vi "module-12-analog-pid-complex.vi"() -> ()   [LabVIEW 2019]
uses:
  <vilib>/Rock Robotics/WPI/ThirdParty/JAS_Junk/TrajLib/PID_CONTROLLER.ctl
  <vilib>/Rock Robotics/WPI/ThirdParty/JAS_Junk/TrajLib/LinearFilter_ResetToValue.vi
  <vilib>/Rock Robotics/WPI/ThirdParty/JAS_Junk/TrajLib/LinearFilter_Calculate.vi
  <vilib>/Rock Robotics/WPI/ThirdParty/JAS_Junk/TrajLib/PIDController_AtSetpoint.vi
  <vilib>/Rock Robotics/WPI/ThirdParty/JAS_Junk/TrajLib/PIDController_SetPIDF.vi
  <vilib>/Rock Robotics/WPI/ThirdParty/JAS_Junk/TrajLib/PIDController_SetDerivativeFilter.vi
  <vilib>/Rock Robotics/WPI/ThirdParty/JAS_Junk/TrajLib/PIDController_SetIntegratorRange.vi
  <vilib>/Rock Robotics/WPI/ThirdParty/JAS_Junk/TrajLib/PIDController_SetTolerancePandV.vi
  <vilib>/Rock Robotics/WPI/ThirdParty/JAS_Junk/TrajLib/PIDController_DisableContinousInput.vi
  <vilib>/Rock Robotics/WPI/ThirdParty/JAS_Junk/TrajLib/PIDController_EnableContinousInput.vi
  <vilib>/Rock Robotics/WPI/ThirdParty/JAS_Junk/TrajLib/PIDController_Reset.vi
  <vilib>/Rock Robotics/WPI/ThirdParty/JAS_Junk/TrajLib/PIDController_New.vi
  <vilib>/Rock Robotics/WPI/ThirdParty/JAS_Junk/TrajLib/PIDController_SetOutputLimits.vi
  <vilib>/Rock Robotics/WPI/ThirdParty/JAS_Junk/TrajLib/ControllerUtil_GetModulusError.vi
  <vilib>/Rock Robotics/WPI/ThirdParty/JAS_Junk/TrajLib/PIDController_NewPeriod.vi
  <vilib>/Rock Robotics/SystemInterfaces/NetworkCommunication/NetComm_UsageReport_report.vi
  <vilib>/addons/control/pid/pid.llb/PID Lead-Lag (DBL).vi
  <vilib>/Rock Robotics/WPI/ThirdParty/JAS_Junk/TrajLib/Util_LibraryGlobals.vi
  <vilib>/Rock Robotics/WPI/ThirdParty/JAS_Junk/TrajLib/PIDController_AdvCalculate_FF_Sp_Pv.vi
  <vilib>/Rock Robotics/WPI/ThirdParty/JAS_Junk/TrajLib/LinearFilter_MovingAverage.vi
  <vilib>/Rock Robotics/WPI/ThirdParty/JAS_Junk/TrajLib/LinearFilter_LowPassBW1.vi
  <vilib>/Rock Robotics/WPI/ThirdParty/JAS_Junk/TrajLib/LinearFilter_LowPassBW2.vi
  <vilib>/Rock Robotics/WPI/ThirdParty/JAS_Junk/TrajLib/LinearFilter_HighPassBW1.vi
  <vilib>/Rock Robotics/WPI/ThirdParty/JAS_Junk/TrajLib/LinearFilter_HighPassBW2.vi
  <vilib>/addons/control/pid/NI_PID_pid.lvlib
  <vilib>/Rock Robotics/WPI/ThirdParty/JAS_Junk/TrajLib/Trajectory_Library.lvlib
panel:
  in  "Tab Control":T1(tab)
  in  "Enable Noise":bool=TRUE
  in  "Auto / Manual":bool=TRUE
  out "Selected Speed Demand":dbl format="%10.2f"
  in  "Desired Speed":dbl(slide)=-0.22222222222222499 scale=-50.0..50.0 scale format="%#.1f"
  out "Selected Speed Target":dbl format="%10.2f"
  out "Right Motor Demand":dbl format="%11.3f"
  out "Right Wheel Speed":dbl(knob)=-2.895988890827539e-05 scale=-60.0..60.0
  out "Right Wheel Error":dbl format="%11.3f"
  out "Right Wheel Speed":dbl format="%10.2f"
  out "Left Wheel Speed":dbl(knob)=-2.895988890827539e-05 scale=-60.0..60.0
  out "Left Wheel Error":dbl format="%11.3f"
  out "Left Motor Demand":dbl format="%11.3f"
  out "Left Wheel Speed":dbl format="%10.2f"
  in  "MinOutput 2":dbl=-9.9e+32
  in  "MaxOutput 2":dbl=9.9e+32
  in  "MinInput 2":dbl
  in  "MaxInput 2":dbl
  in  "MinOutput":dbl=-9.9e+32
  in  "MaxOutput":dbl=9.9e+32
  in  "MinInput":dbl
  in  "MaxInput":dbl
  in  "SetPoint Change Rate":dbl=80.0 min=1.0 max=9000.0 format="%14.4f"
  in  "Right-Kp":dbl=0.12
  in  "Right-Ki":dbl=1.2
  in  "Right-Kd":dbl
  in  "Right-Max-I":dbl=1.0
  in  "Right-Min-I":dbl=-1.0
  in  "Right-Kf":dbl=0.02
  in  "Left-Kp":dbl=0.12
  in  "Left-Ki":dbl=1.2
  in  "Left-Kd":dbl
  in  "Left-Max-I":dbl=1.0
  in  "Left-Min-I":dbl=-1.0
  in  "Left-Kf":dbl=0.02
  out "Right-PID Data":T2={"Kp"=0.0, "Ki"=0.0, "Kd"=0.0, "Period"=0.0, "Max_Integral"=0.0, "Min_Integral"=0.0, "Max_Input"=0.0, "Min_Input"=0.0, "Continuous"=FALSE, "PositionError"=0.0, "VelocityError"=0.0, "PrevError"=0.0, "TotalError"=0.0, "PositionTolerance"=0.0, "VelocityTolerance"=0.0, "SetPoint"=0.0, "Kf"=0.0, "Prev_Deriv"=0.0, "Prev_Deriv 2"=0.0, "DerivativeFilter"=FALSE, "Min_Output"=-9.99e+35, "Max_Output"=9.9e+35, "Prev_F_P"=0.0, "Prev_F_P_2"=0.0, "AntiWindupActive"=FALSE, "Measurement"=0.0} {"Measurement" format="%16_6e"; "Prev_F_P_2" format="%16_6e"; "Prev_F_P" format="%16_6e"; "Max_Output" format="%16_6e"; "Min_Output" format="%16_6e"; "Prev_Deriv 2" format="%16_6e"; "Prev_Deriv" format="%16_6e"; "Kf" format="%16_6e"; "SetPoint" format="%16_6e"; "VelocityTolerance" format="%16_6e"; "PositionTolerance" format="%16_6e"; "TotalError" format="%16_6e"; "PrevError" format="%16_6e"; "VelocityError" format="%16_6e"; "PositionError" format="%16_6e"; "Min_Input" format="%16_6e"; "Max_Input" format="%16_6e"; "Min_Integral" format="%16_6e"; "Max_Integral" format="%16_6e"; "Period" format="%16_6e"; "Kd" format="%16_6e"; "Ki" format="%16_6e"; "Kp" format="%16_6e"}
  out "Left-PID Data":T2={"Kp"=0.0, "Ki"=0.0, "Kd"=0.0, "Period"=0.0, "Max_Integral"=0.0, "Min_Integral"=0.0, "Max_Input"=0.0, "Min_Input"=0.0, "Continuous"=FALSE, "PositionError"=0.0, "VelocityError"=0.0, "PrevError"=0.0, "TotalError"=0.0, "PositionTolerance"=0.0, "VelocityTolerance"=0.0, "SetPoint"=0.0, "Kf"=0.0, "Prev_Deriv"=0.0, "Prev_Deriv 2"=0.0, "DerivativeFilter"=FALSE, "Min_Output"=-9.99e+35, "Max_Output"=9.9e+35, "Prev_F_P"=0.0, "Prev_F_P_2"=0.0, "AntiWindupActive"=FALSE, "Measurement"=0.0} {"Measurement" format="%16_6e"; "Prev_F_P_2" format="%16_6e"; "Prev_F_P" format="%16_6e"; "Max_Output" format="%16_6e"; "Min_Output" format="%16_6e"; "Prev_Deriv 2" format="%16_6e"; "Prev_Deriv" format="%16_6e"; "Kf" format="%16_6e"; "SetPoint" format="%16_6e"; "VelocityTolerance" format="%16_6e"; "PositionTolerance" format="%16_6e"; "TotalError" format="%16_6e"; "PrevError" format="%16_6e"; "VelocityError" format="%16_6e"; "PositionError" format="%16_6e"; "Min_Input" format="%16_6e"; "Max_Input" format="%16_6e"; "Min_Integral" format="%16_6e"; "Max_Integral" format="%16_6e"; "Period" format="%16_6e"; "Kd" format="%16_6e"; "Ki" format="%16_6e"; "Kp" format="%16_6e"}
  in  "RightWheelNoise":dbl
  in  "LeftWheelNoise":dbl
  in  "RightWheelSpeed":dbl
  in  "LeftWheelSpeed":dbl
  in  "RightMotorOutput":dbl
  in  "LeftMotorOutput":dbl
  in  "SpeedSetpoint":dbl
  in  "SpeedTarget":dbl
  in  "SpeedControlEnabled":bool
  out "SP, PV, CO Right":T3(graph)
  out "SP, PV, CO Left":T3(graph)
  # "Example of Closed Loop \nMotor Speed Control"
  # "Enter a desired speed and then press the Set Speed Target \nbutton.  This simulates the joystick input."
  # "This value shows the current speed of each wheel.  This is measured by an encoder.  The encoder measures\n speed by counting pulses of the wheel turning and dividing by the time interval.  Total distance change\nis also a result.  This value is called the \"Process Variable\"."
  # "FT/SEC"
  # "FT/SEC"
  # "FT/SEC"
  # "FT/SEC"
  # "The Speed Target is rate limited so not to make\nto drastic a change in the desired speed.  (This is\nwhat happens mechanically when pushing the gas\npedal of a real car.)"
  # "This error value shows the error between the current speed\nand the speed demand."
  # "FT/SEC"
  # "This example adds a \"Manual\" mode so that the still operates\nif the encoder fails."
  # "FT/SEC"
  # "FT/SEC"
  # "This value shows the current motor output demand.  This could also be a motor speed demand and \nanother closed loop controller would control the motor speed.  In this simple example this value is \nused to drive the simulated motor directly.  This motor demand is called the \"Control Output\"."
  # "Enables some simulated process noise"
  # "FT/SEC/SEC"
  # "These are the tuning parameters for the PID VI"
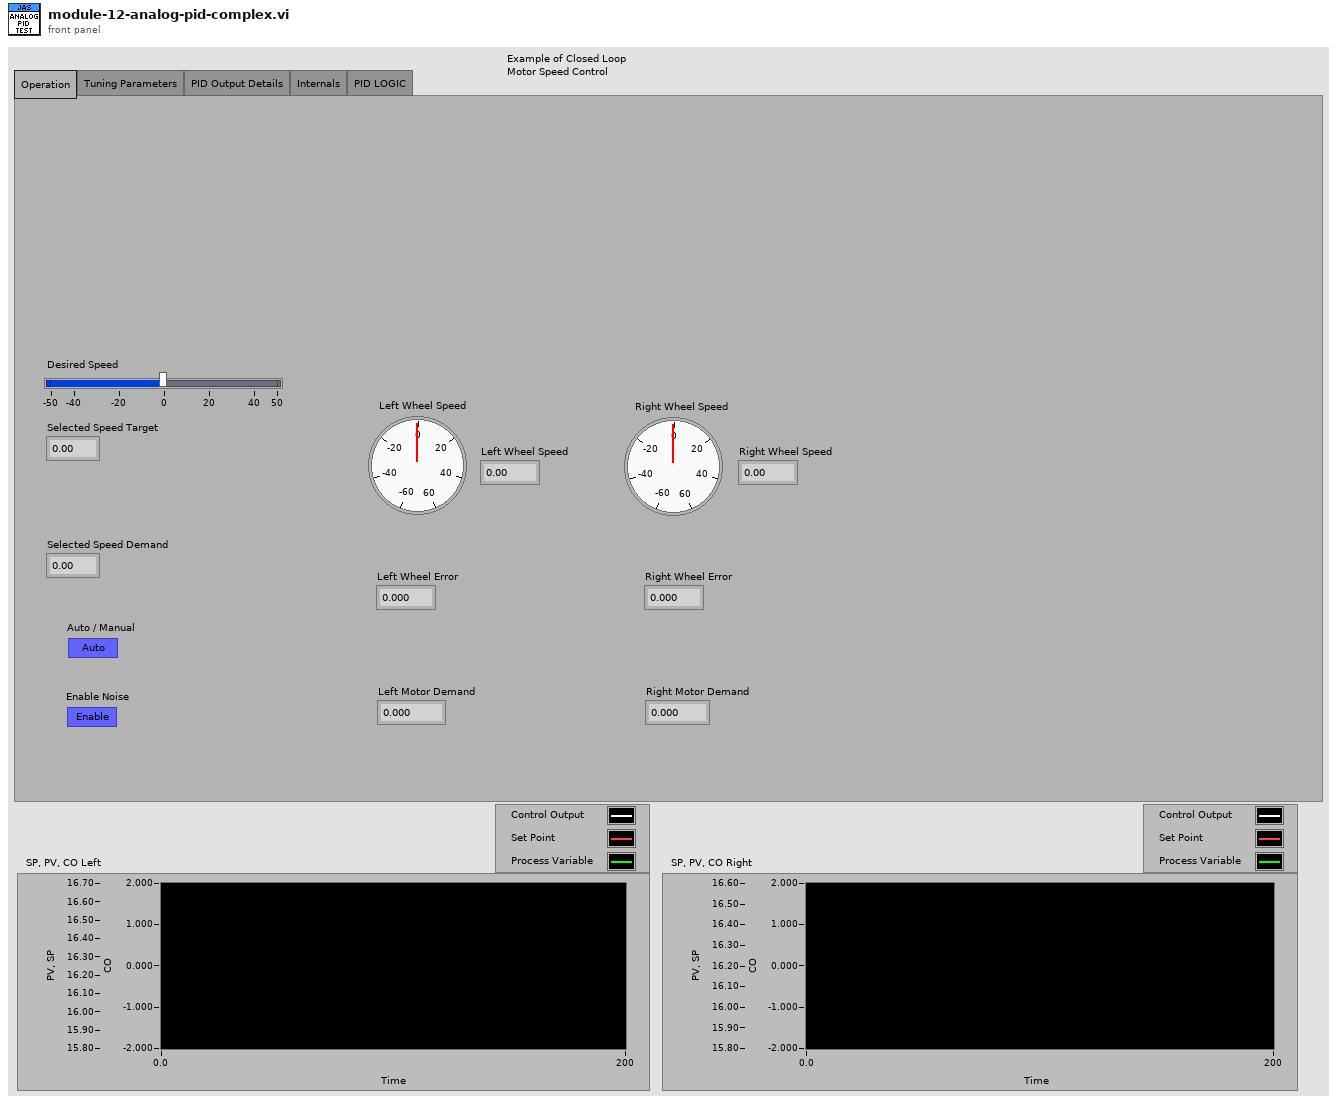
[diagram p1: front panel]
types:
  T1 = enum32{"Operation", "Tuning Parameters", "PID Output Details", "Internals", "PID LOGIC"}
  T2 = typedef "Trajectory_Library.lvlib/PID_CONTROLLER.ctl" = cluster{"Kp":dbl, "Ki":dbl, "Kd":dbl, "Period":dbl, "Max_Integral":dbl, "Min_Integral":dbl, "Max_Input":dbl, "Min_Input":dbl, "Continuous":bool, "PositionError":dbl, "VelocityError":dbl, "PrevError":dbl, "TotalError":dbl, "PositionTolerance":dbl, "VelocityTolerance":dbl, "SetPoint":dbl, "Kf":dbl, "Prev_Deriv":dbl, "Prev_Deriv 2":dbl, "DerivativeFilter":bool, "Min_Output":dbl, "Max_Output":dbl, "Prev_F_P":dbl, "Prev_F_P_2":dbl, "AntiWindupActive":bool, "Measurement":dbl}
  T3 = cluster{"MotorDemand":dbl, "CurrentSetpoint":dbl, "CurrentPosition":dbl}
  T4 = cluster{"gain":dbl, "lag time":dbl, "lead time":dbl}
  T5 = typedef "Trajectory_Library.lvlib/PID_ADV_LIMITS.ctl" = cluster{"MaxInput":dbl, "MinInput":dbl, "Continuous":bool, "MaxOutput":dbl, "MinOutput":dbl}
  T6 = enum16{"Moving Average", "Low Pass 1st Order Butterworth", "Low Pass 2nd Order Butterworth", "High Pass 1st Order Butterworth", "High Pass 2nd Order Butterworth"}
  T7 = cluster{"LeftMotorOutput":dbl, "SpeedSetpoint":dbl, "LeftWheelSpeed":dbl}
  T8 = cluster{"RightMotorOutput":dbl, "SpeedSetpoint":dbl, "RightWheelSpeed":dbl}
  T9 = typedef "Trajectory_Library.lvlib/PID_ADV_TUNING.ctl" = cluster{"Kf":dbl, "Kp":dbl, "Ki":dbl, "Kd":dbl, "MaximumIntegral":dbl, "MinimumIntegral":dbl, "Filter Derivative":bool}
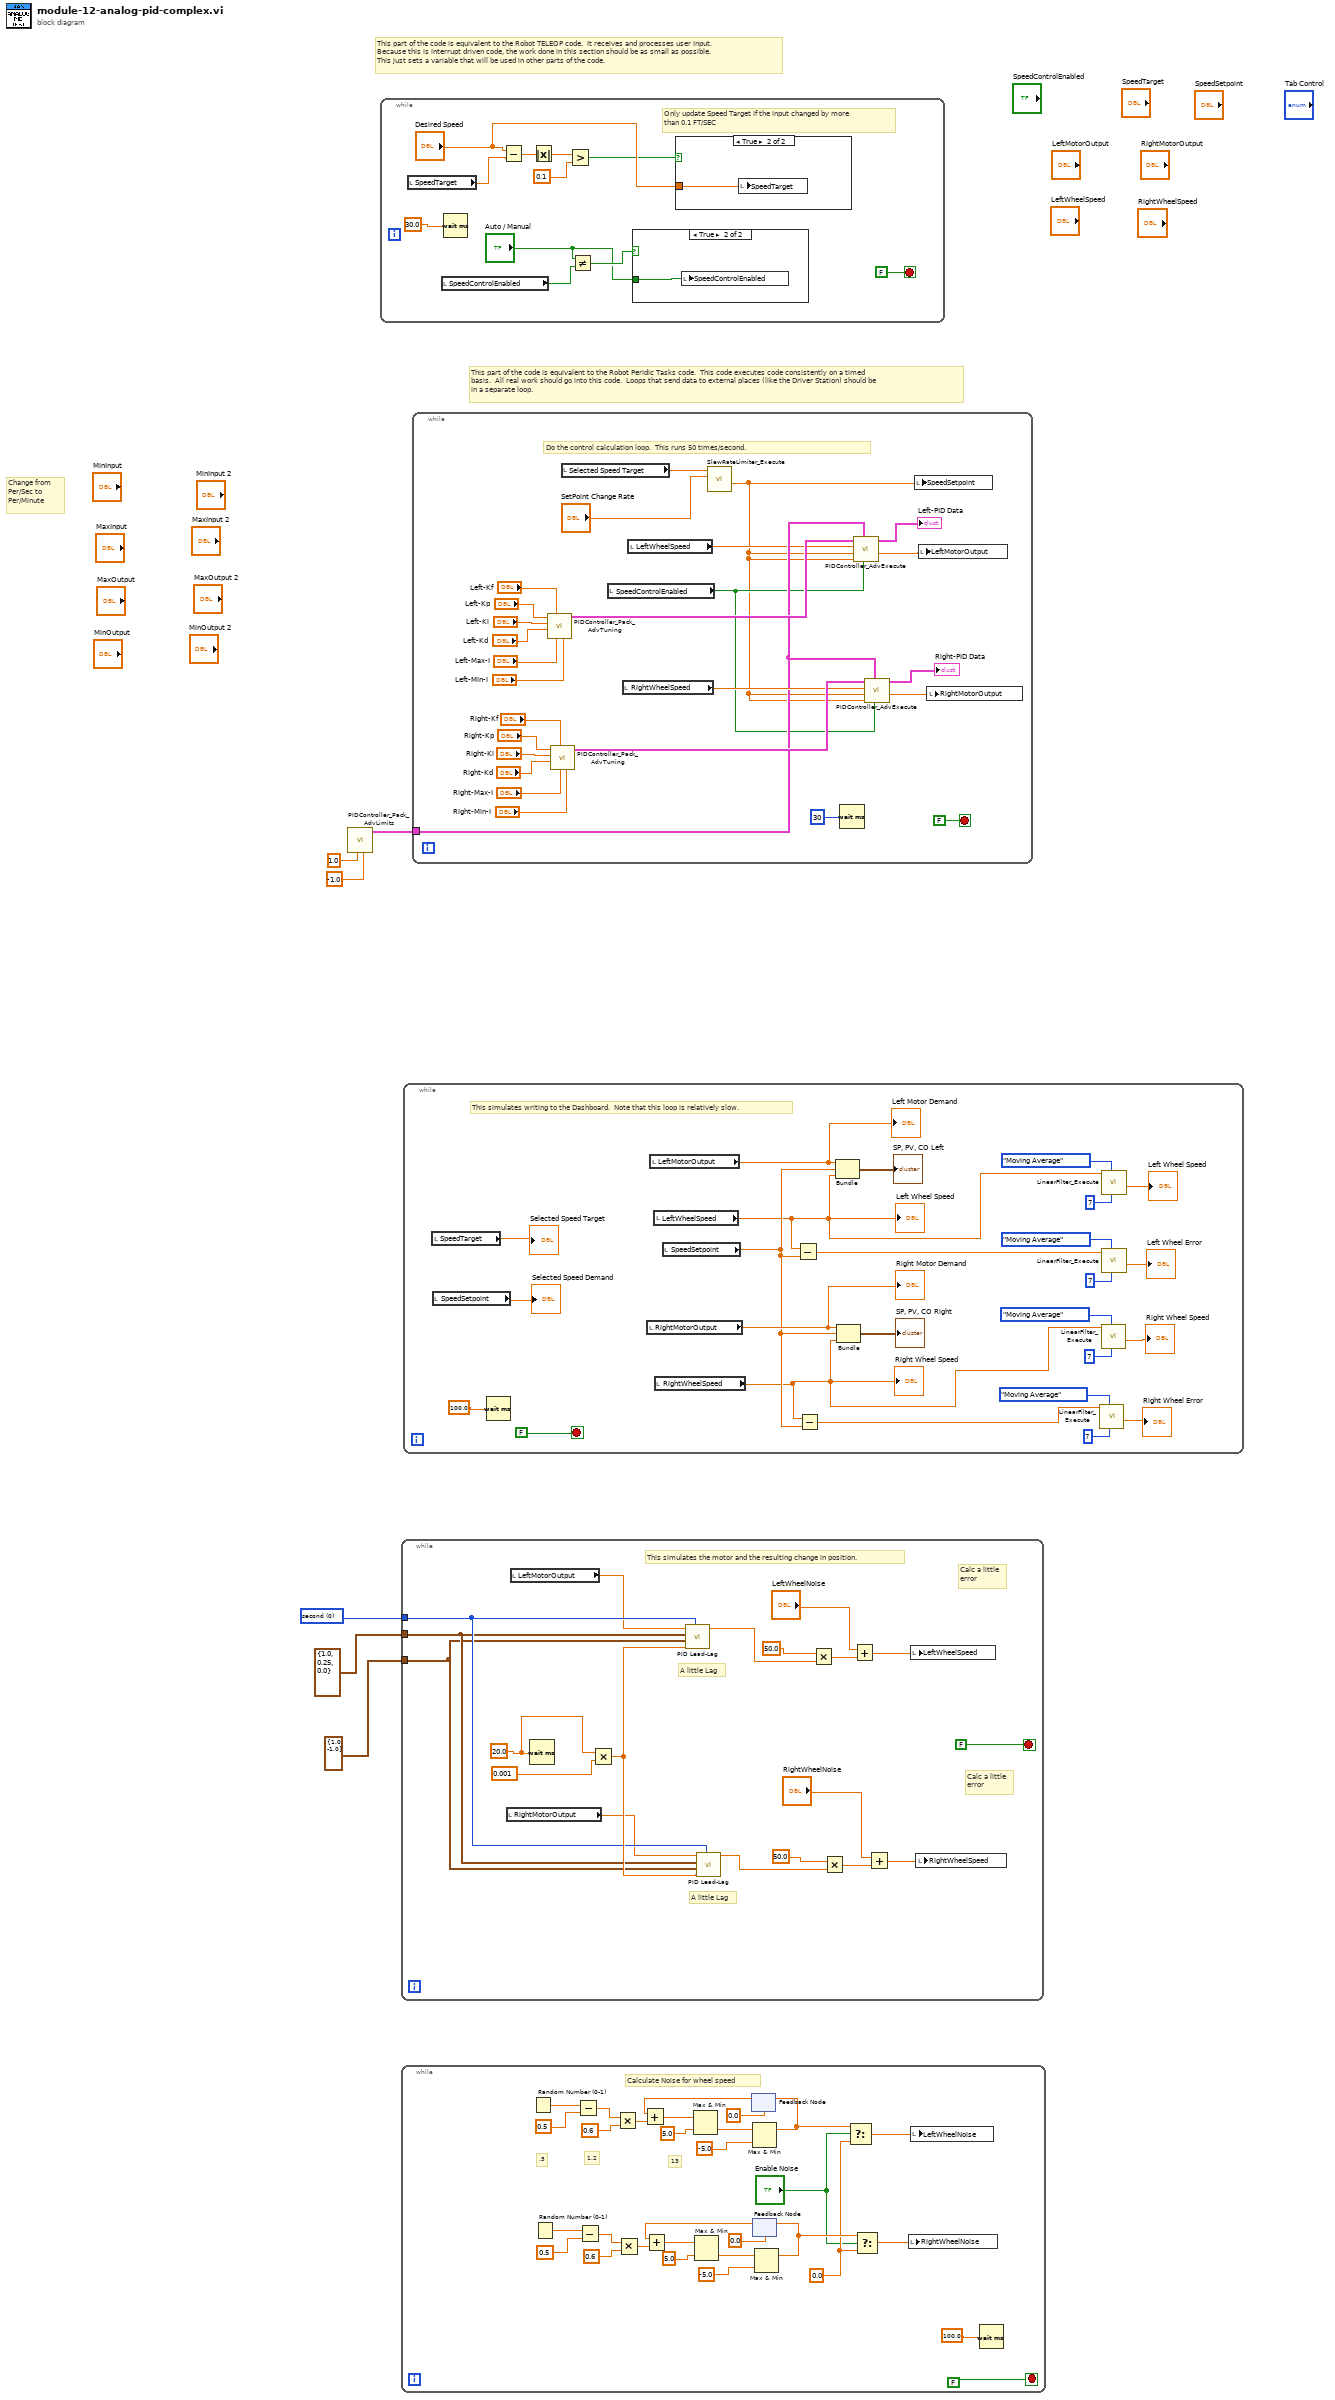
[diagram p0: block diagram]
diagram:
  w6 = u16 0 items=["second", "minute"] ("time unit")
  # "Change from\nPer/Sec to\nPer/Minute"
  # "This part of the code is equivalent to the Robot Peridic Tasks code.  This code executes code consistently on a timed\nbasis.  All real work should go into this code.  Loops that send data to external places (like the Driver Station) should be \nin a separate loop."
  # "This part of the code is equivalent to the Robot TELEOP code.  It receives and processes user input.\nBecause this is interrupt driven code, the work done in this section should be as small as possible.\nThis just sets a variable that will be used in other parts of the code."
  n1 = call <vilib>:"PIDController_Pack_AdvLimits.vi"("MinOutput"=-1.0, "MaxOutput"=1.0) -> ("Adv PID Limits"=w1:T5)  [unwired: 9 in]
  n2 = while {
    stop <- FALSE stop-if-true
    # "Only update Speed Target if the input changed by more\nthan 0.1 FT/SEC"
    n3 = local read "SpeedTarget"() -> (w16:dbl)
    n4 = local read "SpeedControlEnabled"() -> (w8:bool)
    n5 = Wait (ms)(milliseconds to wait=30.0) -> ()  [unwired: 1 out]
    n6 = Subtract(x="Desired Speed", y=w16) -> (x-y=w15:dbl)
    n7 = Absolute Value(x=w15) -> (abs(x)=w14:dbl)
    n8 = Greater?(x=w14, y=0.1) -> (0:w11:bool)
    n9 = Not Equal?(x="Auto / Manual", y=w8) -> (x != y?=w9:bool)
    n10 = case shown="True" w9 {
      tunnel: "Auto / Manual" -> [_ w18]
      frame False {
      }
      frame True {
        n11 = local write "SpeedControlEnabled"(w18) -> ()
      }
    }
    n12 = case shown="True" w11 {
      tunnel: "Desired Speed" -> [_ w19]
      frame False {
      }
      frame True {
        n13 = local write "SpeedTarget"(w19) -> ()
      }
    }
  }
  n14 = while {
    tunnel: w6 -> [w31]
    tunnel: T4 {"gain"=1.0, "lag time"=0.25, "lead time"=0.0} ("tuning parameters") -> [w30]
    tunnel: cluster{"output high":dbl, "output low":dbl} {"output high"=1.0, "output low"=-1.0} ("output range") -> [w29]
    stop <- FALSE stop-if-true
    w35 = 20.0
    # "This simulates the motor and the resulting change in position."
    # "Calc a little\nerror"
    # "Calc a little\nerror"
    # "A little Lag"
    # "A little Lag"
    n15 = local read "RightMotorOutput"() -> (w22:dbl)
    n16 = local read "LeftMotorOutput"() -> (w25:dbl)
    n17 = Wait (ms)(milliseconds to wait=w35) -> ()  [unwired: 1 out]
    n18 = Multiply(x=w35, y=0.001) -> (x*y=w32:dbl)
    n19 = call-poly <vilib>:"PID Lead-Lag.vi"("time unit"=w31, "dt (s)"=w32, "output range"=w29, "tuning parameters"=w30, "input"=w25) -> ("output"=w34:dbl)  [unwired: 3 in, 1 out]
    n20 = call-poly <vilib>:"PID Lead-Lag.vi"("time unit"=w31, "dt (s)"=w32, "output range"=w29, "tuning parameters"=w30, "input"=w22) -> ("output"=w26:dbl)  [unwired: 3 in, 1 out]
    n21 = Multiply(x=50.0, y=w34) -> (x*y=w27:dbl)
    n22 = Multiply(x=50.0, y=w26) -> (x*y=w28:dbl)
    n23 = Add(x="LeftWheelNoise", y=w27) -> (x+y=w24:dbl)
    n24 = Add(x="RightWheelNoise", y=w28) -> (x+y=w23:dbl)
    n25 = local write "LeftWheelSpeed"(w24) -> ()
    n26 = local write "RightWheelSpeed"(w23) -> ()
  }
  n27 = while {
    stop <- FALSE stop-if-true
    w40 = 0.0 ("f")
    # "Calculate Noise for wheel speed"
    # "13"
    # "1.2"
    # ".5"
    n28 = Random Number (0-1)() -> (number: 0 to 1=w66:dbl)
    n29 = Random Number (0-1)() -> (number: 0 to 1=w55:dbl)
    n30 = Subtract(x=w66, y=0.5) -> (x-y=w58:dbl)
    n31 = Subtract(x=w55, y=0.5) -> (x-y=w47:dbl)
    n32 = Multiply(x=w58, y=0.6) -> (x*y=w57:dbl)
    n33 = Multiply(x=w47, y=0.6) -> (x*y=w46:dbl)
    n34 = feedback #1(0.0) -> (w60:dbl)
    n35 = Add(x=w60, y=w57) -> (x+y=w64:dbl)
    n36 = Max & Min(x=w64, y=5.0) -> (min(x,y)=w63:dbl)  [unwired: 1 out]
    n37 = Max & Min(x=w63, y=-5.0) -> (max(x,y)=w43:dbl)  [unwired: 1 out]
    n38 = feedback-in #1(w43) -> ()
    n39 = feedback #2(0.0) -> (w49:dbl)
    n40 = Add(x=w49, y=w46) -> (x+y=w53:dbl)
    n41 = Max & Min(x=w53, y=5.0) -> (min(x,y)=w52:dbl)  [unwired: 1 out]
    n42 = Max & Min(x=w52, y=-5.0) -> (max(x,y)=w41:dbl)  [unwired: 1 out]
    n43 = feedback-in #2(w41) -> ()
    n44 = Select(t=w43, s="Enable Noise", f=w40) -> (s? t:f=w44:dbl)
    n45 = Select(t=w41, s="Enable Noise", f=w40) -> (s? t:f=w42:dbl)
    n46 = local write "RightWheelNoise"(w42) -> ()
    n47 = local write "LeftWheelNoise"(w44) -> ()
    n48 = Wait (ms)(milliseconds to wait=100.0) -> ()  [unwired: 1 out]
  }
  n49 = while {
    stop <- FALSE stop-if-true
    # "This simulates writing to the Dashboard.  Note that this loop is relatively slow."
    n50 = local read "SpeedTarget"() -> (→"Selected Speed Target":dbl)
    n51 = local read "SpeedSetpoint"() -> (→"Selected Speed Demand":dbl)
    n52 = Wait (ms)(milliseconds to wait=100.0) -> ()  [unwired: 1 out]
    n53 = local read "RightMotorOutput"() -> (w89:dbl)
    "Right Motor Demand" <- w89
    n54 = local read "LeftMotorOutput"() -> (w86:dbl)
    "Left Motor Demand" <- w86
    n55 = local read "LeftWheelSpeed"() -> (w73:dbl)
    "Left Wheel Speed" <- w73
    n56 = local read "RightWheelSpeed"() -> (w76:dbl)
    "Right Wheel Speed" <- w76
    n57 = local read "SpeedSetpoint"() -> (w85:dbl)
    n58 = Subtract(x=w73, y=w85) -> (x-y=w74:dbl)
    n59 = Subtract(x=w76, y=w85) -> (x-y=w75:dbl)
    n60 = Bundle("LeftMotorOutput"=w86, "SpeedSetpoint"=w85, "LeftWheelSpeed"=w73) -> (→"SP, PV, CO Left":T7)  [unwired: 1 in]
    n61 = Bundle("RightMotorOutput"=w89, "SpeedSetpoint"=w85, "RightWheelSpeed"=w76) -> (→"SP, PV, CO Right":T8)  [unwired: 1 in]
    n62 = call <vilib>:"LinearFilter_Execute.vi"("Samples"=7, "Filter Type"=T6."Moving Average", "Input"=w75) -> ("Output"=→"Right Wheel Error":dbl)  [unwired: 7 in, 1 out]
    n63 = call <vilib>:"LinearFilter_Execute.vi"("Samples"=7, "Filter Type"=T6."Moving Average", "Input"=w76) -> ("Output"=→"Right Wheel Speed":dbl)  [unwired: 7 in, 1 out]
    n64 = call <vilib>:"LinearFilter_Execute.vi"("Samples"=7, "Filter Type"=T6."Moving Average", "Input"=w73) -> ("Output"=→"Left Wheel Speed":dbl)  [unwired: 7 in, 1 out]
    n65 = call <vilib>:"LinearFilter_Execute.vi"("Samples"=7, "Filter Type"=T6."Moving Average", "Input"=w74) -> ("Output"=→"Left Wheel Error":dbl)  [unwired: 7 in, 1 out]
  }
  n66 = while {
    tunnel: w1 -> [w99]
    stop <- FALSE stop-if-true
    # "Do the control calculation loop.  This runs 50 times/second."
    n67 = call <vilib>:"PIDController_Pack_AdvTuning.vi"("MinimumIntegral"="Left-Min-I", "MaximumIntegral"="Left-Max-I", "Kf"="Left-Kf", "Kd"="Left-Kd", "Ki"="Left-Ki", "Kp"="Left-Kp") -> ("Adv PID Tuning"=w102:T9)  [unwired: 5 in]
    n68 = call <vilib>:"PIDController_Pack_AdvTuning.vi"("MinimumIntegral"="Right-Min-I", "MaximumIntegral"="Right-Max-I", "Kf"="Right-Kf", "Kd"="Right-Kd", "Ki"="Right-Ki", "Kp"="Right-Kp") -> ("Adv PID Tuning"=w113:T9)  [unwired: 5 in]
    n69 = local read "Selected Speed Target"() -> (w95:dbl)
    n70 = local read "SpeedControlEnabled"() -> (w97:bool)
    n71 = local read "RightWheelSpeed"() -> (w110:dbl)
    n72 = local read "LeftWheelSpeed"() -> (w98:dbl)
    n73 = call <vilib>:"SlewRateLimiter_Execute.vi"("Rate"="SetPoint Change Rate", "Input"=w95) -> ("Output"=w96:dbl)  [unwired: 8 in, 1 out]
    n74 = Wait (ms)(milliseconds to wait=u32 30) -> ()  [unwired: 1 out]
    n75 = call <vilib>:"PIDController_AdvExecute.vi"("Auto"=w97, "Adv PID Limits"=w99, "FF-FeedForward"=w96, "SP-SetPoint"=w96, "PV-Measurement"=w98, "Adv PID Tuning"=w102) -> ("CO-ControlOutput"=w101:dbl, "out PID_CONTROLLER"=→"Left-PID Data":T2)  [unwired: 3 in, 1 out]
    n76 = call <vilib>:"PIDController_AdvExecute.vi"("Auto"=w97, "Adv PID Limits"=w99, "FF-FeedForward"=w96, "SP-SetPoint"=w96, "PV-Measurement"=w110, "Adv PID Tuning"=w113) -> ("CO-ControlOutput"=w109:dbl, "out PID_CONTROLLER"=→"Right-PID Data":T2)  [unwired: 3 in, 1 out]
    n77 = local write "SpeedSetpoint"(w96) -> ()
    n78 = local write "LeftMotorOutput"(w101) -> ()
    n79 = local write "RightMotorOutput"(w109) -> ()
  }
